vi "RSZVB Set Frequency LO Conversion Factor.vi"(6 "Denominator (1)":i32=1, 7 "Numerator (1)":i32=1, 8 "error in (no error)":errorcluster {"code" format="%.0x"}, 9 "Stage (1)":i32=1, 10 "Channel (1)":i32=1, 11 "VISA resource name":refnum<visa-resource-name>) -> (0 "error out":errorcluster {"code" format="%.0x"}, 3 "VISA resource name out":refnum<visa-resource-name>)   [LabVIEW 2011]
doc: "This VI sets the frequency conversion factors for the LO 1 or L0 2 signal.\n\nRemote-control command(s):\n[SENSe<Ch>:]FREQuency:CONVersion:MIXer:LOMultiplier<Stg> <numerator>,<denominator>"
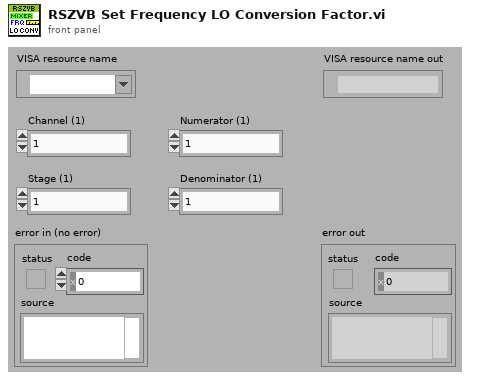
[diagram p1: front panel]
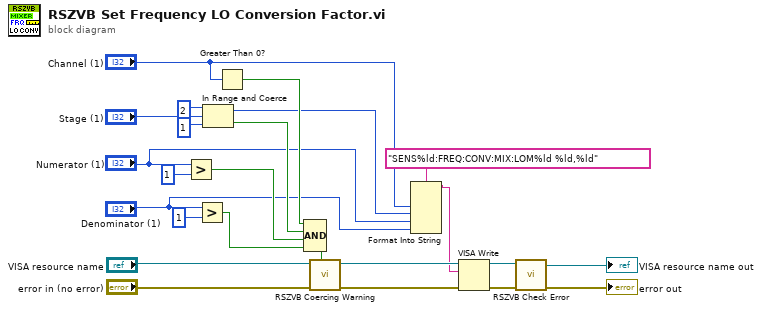
[diagram p0: block diagram]
diagram:
  n1 = Greater?(x="Numerator (1)", y=1) -> (0:w6:bool)
  n2 = Greater?(x="Denominator (1)", y=1) -> (0:w7:bool)
  n3 = In Range and Coerce(upper limit=2, x="Stage (1)", lower limit=1) -> (coerced(x)=w5:i32, In Range?=w10:bool)
  n4 = Greater Than 0?(x="Channel (1)") -> (x > 0?=w12:bool)
  n5 = Compound Arithmetic op=AND(w12, w10, w6, w7) -> (w20:bool)
  n6 = call "RSZVB Coercing Warning.vi"("In Range?"=w20, "error in (no error)"="error in (no error)", "VISA session"="VISA resource name") -> ("error out"=w23:errorcluster, "dup VISA session"=w24:refnum<visa-resource-name>)  [unwired: 7 in]
  n7 = Format Into String(format string="SENS%ld:FREQ:CONV:MIX:LOM%ld %ld,%ld", "Channel (1)", w5, "Numerator (1)", "Denominator (1)") -> (resulting string=w18:string)  [unwired: 2 in, 1 out]
  n8 = VISA Write(VISA resource name=w24, write buffer=w18, error in (no error)=w23) -> (VISA resource name out=w21:refnum<visa-resource-name>, error out=w22:errorcluster)  [unwired: 1 out]
  n9 = call "RSZVB Check Error.vi"("error in (no error)"=w22, "VISA session"=w21) -> ("error out"=→"error out":errorcluster, "dup VISA session"=→"VISA resource name out":refnum<visa-resource-name>)  [unwired: 8 in]
